vi "PV ActiveLine - Ethernet.vi"(0 "Referenz in":refnum<visa-resource-name>, 1 "W/R":bool, 5 "ip type (DHCP)":bool, 7 "fixed ip":string, 9 "subnet mask":string, 11 "Fehler (Eingang)":errorcluster, 12 "gateway":string) -> (4 "Referenz out":refnum<visa-resource-name>, 6 "ip type (DHCP) out":bool, 8 "fixed ip out":string, 10 "subnet mask out":string, 14 "gateway out":string, 15 "Cluster (Ausgang)":errorcluster caption="Fehler (Ausgang)")   [LabVIEW 2013, in "PV ActiveLine.lvlib"]
doc: "ETH - Ethernet Configuration\n\nReceive: a,bbb.bbb.bbb.bbb,ccc.ccc.ccc.ccc,ddd.ddd.ddd.ddd\n\nDHCP (dynamic host configuration protocol),\na =\n0 –> Statically\n1 –> Dynamically\nbbb.bbb.bbb.bbb = IP address\nccc.ccc.ccc.ccc = Subnet address\nddd.ddd.ddd.ddd = Gateway address"
uses:
  <instrlib>/PV ActiveLine/PV ActiveLine.lvlib
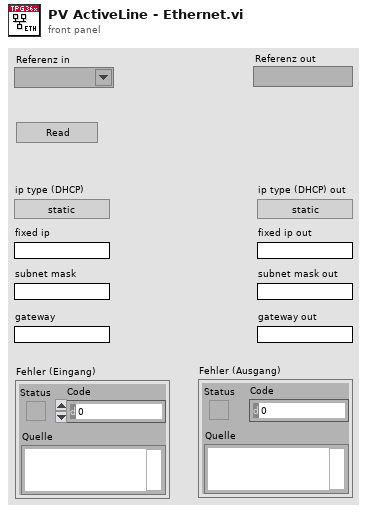
[diagram p1: front panel]
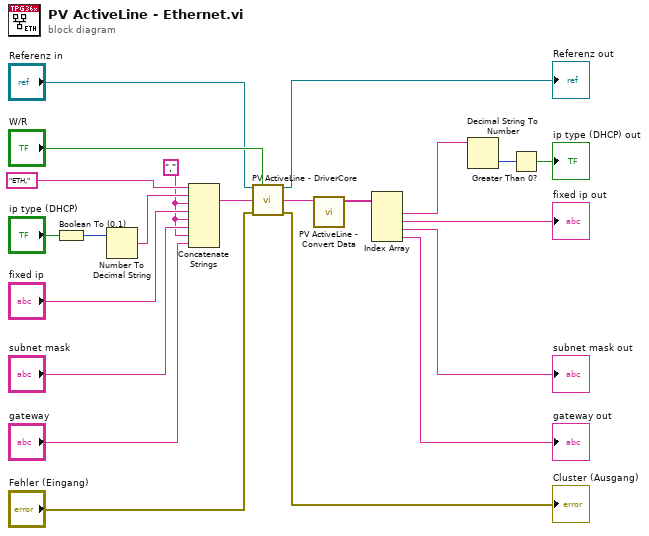
[diagram p0: block diagram]
diagram:
  w12 = "," ("string")
  n1 = Boolean To (0,1)(Boolean="ip type (DHCP)") -> (0, 1=w16:i16)
  n2 = Number To Decimal String(number=w16) -> (decimal integer string=w15:string)  [unwired: 1 in]
  n3 = Concatenate Strings("ETH,", w15, w12, "fixed ip", w12, "subnet mask", w12, "gateway") -> (w20:string)
  n4 = call <instrlib>:"PV ActiveLine - DriverCore.vi"("Referenz in"="Referenz in", "Write/Read"="W/R", "Command"=w20, "Fehler (Eingang)"="Fehler (Eingang)") -> ("Referenz out"=→"Referenz out":refnum<visa-resource-name>, "String Out"=w7:string, "Cluster (Ausgang)"=→"Cluster (Ausgang)":errorcluster)  [unwired: 9 in]
  n5 = call <instrlib>:"PV ActiveLine - Convert Data.vi"("String in"=w7) -> ("String out"=w6:string[])  [unwired: 7 in, 3 out]
  n6 = Index Array(array=w6) -> (element #1=w5:string, element #2=→"fixed ip out":string, element #3=→"subnet mask out":string, element #4=→"gateway out":string)  [unwired: 4 in]
  n7 = Decimal String To Number(string=w5) -> (number=w1:i32)  [unwired: 2 in, 1 out]
  n8 = Greater Than 0?(x=w1) -> (x > 0?=→"ip type (DHCP) out":bool)
